vi "PID test 1.vi"   [LabVIEW 2009]
types:
  T1 = cluster{"proportional gain (Kc)":dbl, "integral time (Ti, min)":dbl, "derivative time (Td, min)":dbl}
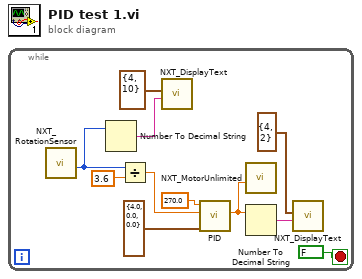
[diagram p0: block diagram]
diagram:
  n1 = while {
    stop <- FALSE stop-if-true
    n2 = call <vilib>:"NXT_RotationSensor.vi"() -> ("Degrees out"=w6:i32)  [unwired: 8 in, 3 out]
    n3 = Number To Decimal String(number=w6) -> (decimal integer string=w4:string)  [unwired: 1 in]
    n4 = Divide(x=w6, y=3.6) -> (x/y=w7:dbl)
    n5 = call <vilib>:"NXT_DisplayText.vi"("Text"=w4, "Location (0,0)"=cluster{"X":i16, "Y":i16} {"X"=4, "Y"=10}) -> ()  [unwired: 9 in, 1 out]
    n6 = call "PID.vi"("coeffecients"=T1 {"proportional gain (Kc)"=4.0, "integral time (Ti, min)"=0.0, "derivative time (Td, min)"=0.0} ("PID gains"), "process variable"=w7, "setpoint"=270.0) -> ("output"=w5:dbl)  [unwired: 7 in, 1 out]
    n7 = call <vilib>:"NXT_MotorUnlimited.vi"("Power (75)"=w5) -> ()  [unwired: 9 in, 2 out]
    n8 = Number To Decimal String(number=w5) -> (decimal integer string=w2:string)  [unwired: 1 in]
    n9 = call <vilib>:"NXT_DisplayText.vi"("Text"=w2, "Location (0,0)"=cluster{"X":i16, "Y":i16} {"X"=4, "Y"=2}) -> ()  [unwired: 9 in, 1 out]
  }
